vi "1. Input Array.vi"() -> ()   [LabVIEW 2012]
panel:
  in  "Column":i32
  in  "Row":i32
  out "Array 2":dbl[][](array[numeric])
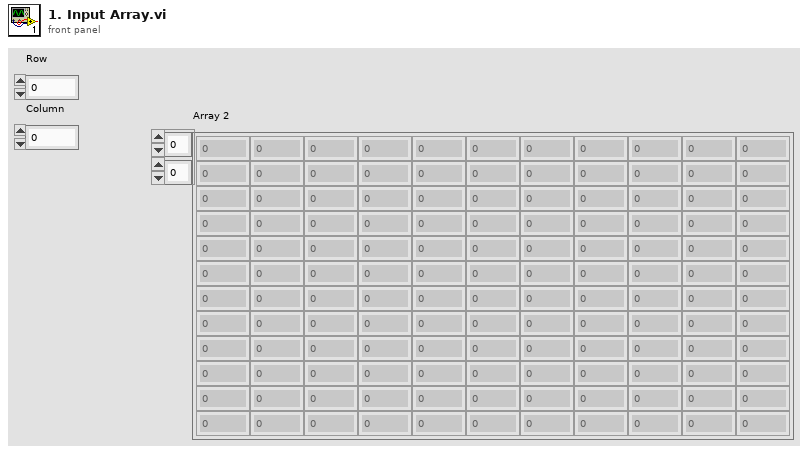
[diagram p1: front panel]
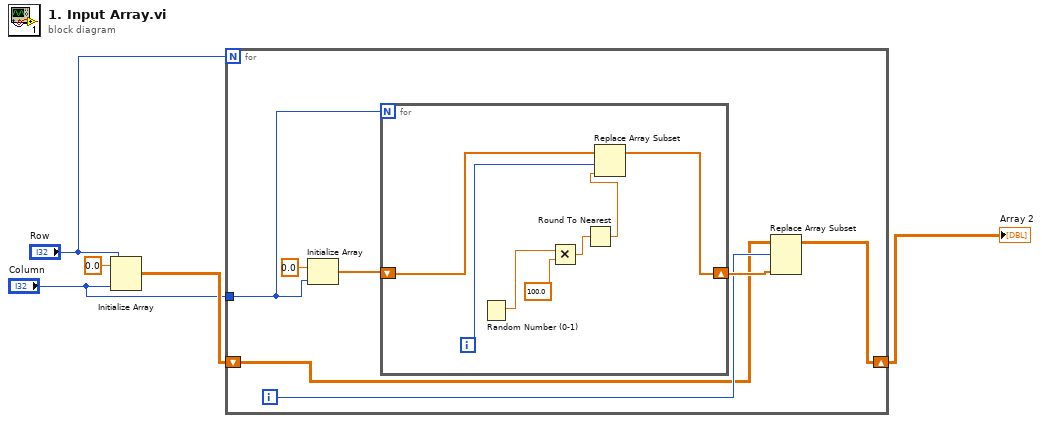
[diagram p0: block diagram]
diagram:
  n1 = Initialize Array(0.0 ("element"), "Row", "Column") -> (w3:dbl[][])
  n2 = for {
    N: "Row" -> [_]
    shift-right: [w9] -> w5
    shift-left: w3 -> [w10]
    tunnel: "Column" -> [w6]
    i -> [w11]
    n3 = Initialize Array(0.0 ("element"), w6) -> (w8:dbl[])
    n4 = for {
      N: w6 -> [_]
      shift-right: [w19] -> w12
      shift-left: w8 -> [w17]
      i -> [w18]
      n5 = Random Number (0-1)() -> (number: 0 to 1=w16:dbl)
      n6 = Multiply(x=w16, y=100.0) -> (x*y=w14:dbl)
      n7 = Round To Nearest(number=w14) -> (nearest integer value=w13:dbl)
      n8 = Replace Array Subset "Replace Array Subset"(array=w17, new element=w13, index=w18) -> (w19:dbl[])
    }
    n9 = Replace Array Subset "Replace Array Subset"(array=w10, new element=w12, index (row)=w11) -> (w9:dbl[][])  [unwired: 1 in]
  }
  "Array 2" <- w5
